vi "Read Display - Units.vi"(8 "error in (no error)":errorcluster, 11 "NT Scalar (Numeric) in":refnum<class "NT Scalar (Numeric).lvclass">) -> (0 "error out":errorcluster, 2 "units":string, 3 "NT Scalar (Numeric) out":refnum<class "NT Scalar (Numeric).lvclass">)   [LabVIEW 2020, in "PV Access.lvlib" / "PV Data.lvlib" / "NT Scalar (Numeric).lvclass"]
uses:
  NT Scalar (Numeric).lvclass
  965e14c5-5dc8-46de-9d5c-d92008508526.vi
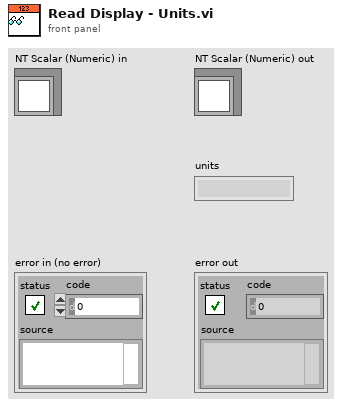
[diagram p1: front panel]
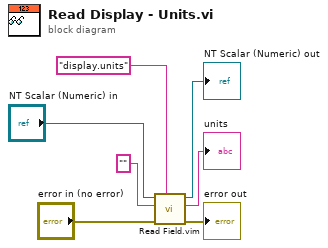
[diagram p0: block diagram]
diagram:
  n1 = call "Read Field.vim"("field"="display.units", "error in"="error in (no error)", "default value"="", "Base Interface in"="NT Scalar (Numeric) in") -> ("error out"=→"error out":errorcluster, "value"=→"units":string, "Base Interface out"=→"NT Scalar (Numeric) out":refnum<class "NT Scalar (Numeric).lvclass">)  [unwired: 5 in]
